vi "Write&ReadAccess3.vi"(8 "error in":errorcluster) -> (0 "error out":errorcluster, 2 "¿Esta abierto?":bool)   [LabVIEW 2019]
doc: "Este VI puede leer y escribir en un documento de Microsoft Word. Se puede switchear entre esta dos opciones en el front panel durante la ejecución"
panel:
  in  "Name":string="Table1"
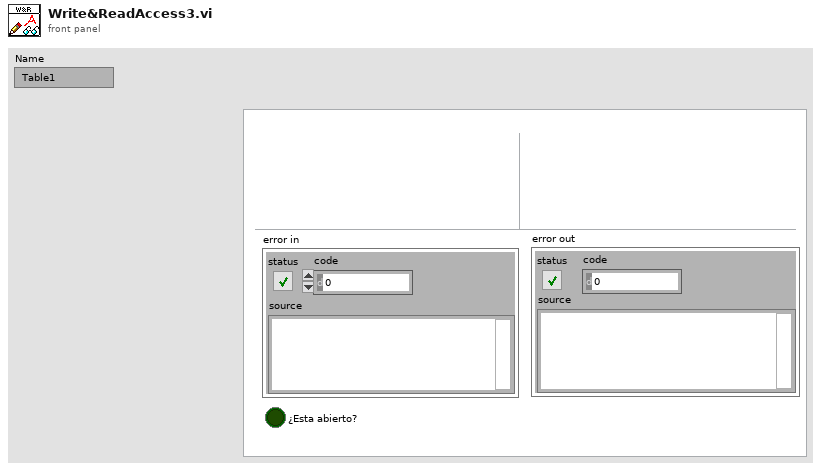
[diagram p1: front panel]
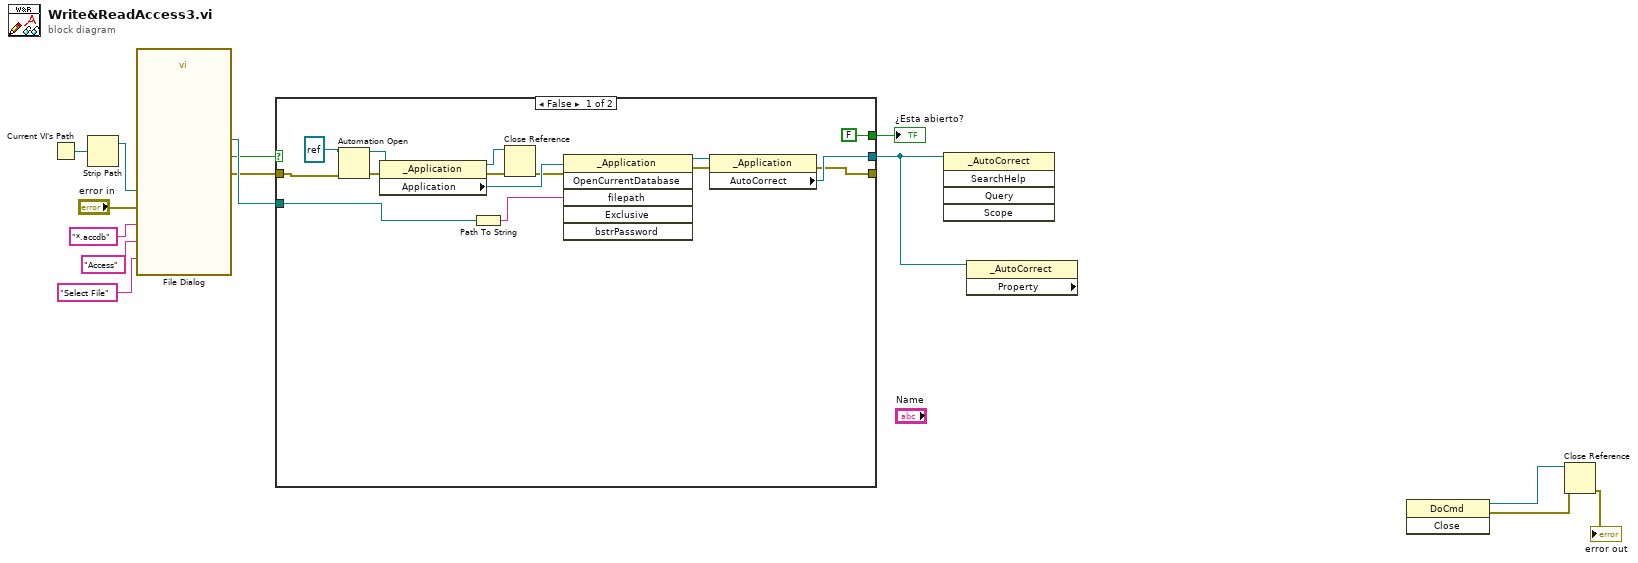
[diagram p0: block diagram]
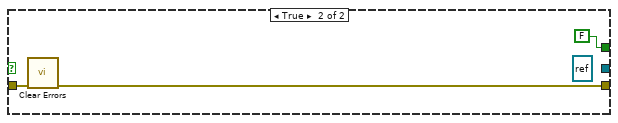
[diagram p2: hidden frame]
diagram:
  n1 = Current VI's Path() -> (path=w12:path)
  n2 = Strip Path(path=w12) -> (stripped path=w14:path)  [unwired: 1 out]
  n3 = call "File Dialog"("start path"=w14, "prompt"="Select File", "error in"="error in", "pattern (all files)"="*.accdb", "pattern label"="Access") -> ("selected path"=w8:path, "cancelled"=w7:bool, "error out"=w6:errorcluster)  [unwired: 7 in, 1 out]
  n4 = case shown="False" w7 {
    tunnel: w8 -> [w29 _]
    tunnel: w6 -> [w25 w32]
    tunnel: [FALSE FALSE] -> w2
    tunnel: [w16 w31] -> _
    tunnel: [w17 _] -> w1
    frame False {
      n5 = Automation Open(error in (no error)=w25, Automation Refnum=refnum<k7> refnum ("Access._Application")) -> (Automation Refnum=w23:refnum<k7>, error out=w22:errorcluster)  [unwired: 2 in]
      n6 = property class="_Application"(reference=w23, error in=w22) -> (reference out=w27:refnum<k7>, error out=w26:errorcluster, "Application"=w21:refnum<k7>)
      n7 = Path To String(path=w29) -> (string=w19:string)
      n8 = Close Reference(reference=w27, error in (no error)=w26) -> (error out=w20:errorcluster)
      n9 = invoke class="_Application" method="OpenCurrentDatabase"(reference=w21, error in=w20, "filepath"=w19) -> (reference out=w15:refnum<k7>, error out=w18:errorcluster)  [unwired: 3 in, 4 out]
      n10 = property class="_Application"(reference=w15, error in=w18) -> (error out=w16:errorcluster, "AutoCorrect"=w17:refnum<k7>)  [unwired: 1 out]
    }
    frame True {
      (unwired) refnum<k7> refnum ("DoCmd")
      n11 = call <vilib>:"Clear Errors.vi"("error in (no error)"=w32) -> ("error out"=w31:errorcluster)  [unwired: 5 in, 1 out]
    }
  }
  "¿Esta abierto?" <- w2
  n12 = invoke class="_AutoCorrect" method="SearchHelp"(reference=w1) -> ()  [unwired: 4 in, 5 out]
  n13 = property class="_AutoCorrect" props=[](reference=w1) -> ()  [unwired: 1 in, 3 out]
  n14 = invoke class="DoCmd" method="Close"() -> (reference out=w4:refnum<k7>, error out=w3:errorcluster)  [unwired: 3 in, 1 out]
  n15 = Close Reference(reference=w4, error in (no error)=w3) -> (error out=→"error out":errorcluster)
